vi "Inverse Time Curve.vi"(6 "error in (no error)":errorcluster, 7 "input cluster":T1={"A [s]"=1.0, "B [s]"=1.0, "alpha"=1.0, "K2 [s]"=1.0, "K1 [s]"=1.0, "K3 [s]"=1.0}, 8 "time dial":dbl=1.0, 9 "multiples of pickup":dbl) -> (0 "error out":errorcluster, 2 "original time":dbl)   [LabVIEW 2016]
uses:
  <vilib>/addons/Electrical Power/Protection/Inverse Time Delay/subVIs/ep_Operate Time.ctl
  <vilib>/addons/Electrical Power/Protection/NI_EP_Protection.lvlib
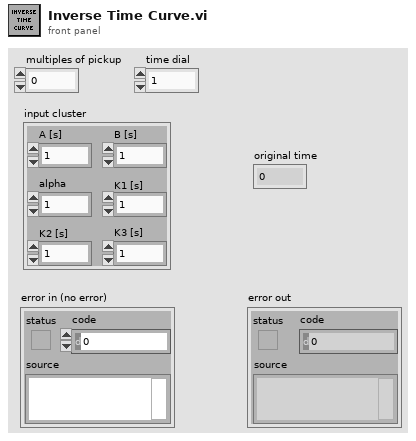
[diagram p1: front panel]
types:
  T1 = typedef "NI_EP_Protection.lvlib/ep_Operate Time.ctl" = cluster{"A [s]":dbl, "B [s]":dbl, "alpha":dbl, "K2 [s]":dbl, "K1 [s]":dbl, "K3 [s]":dbl}
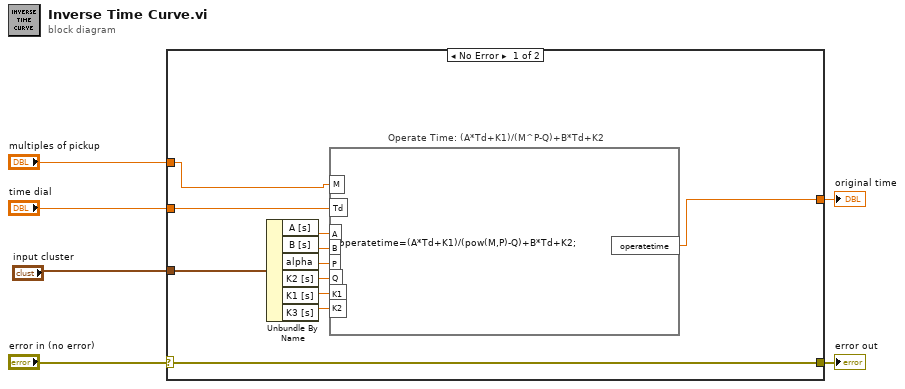
[diagram p0: block diagram]
diagram:
  n1 = case shown="No Error" "error in (no error)" {
    selector: "error in (no error)" -> [w15 w18]
    tunnel: "time dial" -> [w17 _]
    tunnel: "multiples of pickup" -> [w16 _]
    tunnel: [w15 w18] -> w3
    tunnel: [w14 _] -> w2
    tunnel: "input cluster" -> [w7 _]
    frame No Error {
      # "Operate Time: (A*Td+K1)/(M^P-Q)+B*Td+K2"
      n2 = Unbundle By Name(w7) -> ("A [s]"=w13:dbl, "B [s]"=w12:dbl, "alpha"=w11:dbl, "K2 [s]"=w10:dbl, "K1 [s]"=w9:dbl, "K3 [s]"=w8:dbl)
      n3 = formula code="operatetime=(A*Td+K1)/(pow(M,P)-Q)+B*Td+K2;"("A"=w13, "B"=w12, "P"=w11, "Q"=w10, "K1"=w9, "K2"=w8, "Td"=w17, "M"=w16) -> ("operatetime"=w14:dbl)
    }
    frame Error {
    }
  }
  "error out" <- w3
  "original time" <- w2
